vi "open file.vi"(8 "error in (no error)":errorcluster caption="에러 입력(에러 없음)", 10 "file path":path, 11 "Text File 입력":refnum<class "Text File.lvclass">) -> (0 "error out":errorcluster caption="에러 출력", 3 "Text File 출력":refnum<class "Text File.lvclass">)   [LabVIEW 2020, in "Text File.lvclass"]
uses:
  Text File.lvclass
  Haptic IC Class/Haptic IC/Haptic IC.lvclass/Haptic IC.ctl
  Haptic IC Class/Haptic IC/Controls/(Ctrl)IC Type.ctl
  Text File.lvclass/Text File.ctl
  Waveform Obj/Waveform Obj.lvclass/Waveform Obj.ctl
  Accessors/Write Text_File_PWL.vi
  Waveform Obj/Accessors/Write name.vi
  Haptic IC Class/Haptic IC/Accessors/Read ic type.vi
  Waveform Obj/Accessors/Read play mode.vi
  Variables/(Var)System Variables.vi
  Haptic IC Class/Haptic IC/Haptic IC.lvclass
panel:
  in  "TXT_End of LIne":enum16{"EOL (\\r\\n)", "LF (\\n)"}(ring)
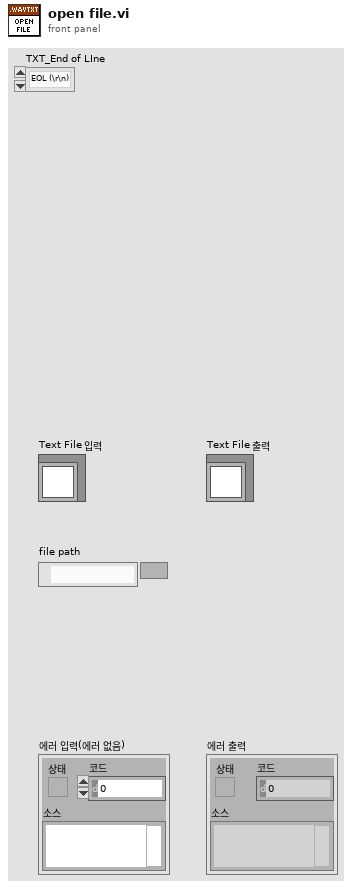
[diagram p1: front panel]
types:
  T1 = cluster{"TXT_Radix":enum16{"BIN", "DEC", "HEX"}, "TXT_Prefix":bool, "TXT_Delimiter":string, "TXT_End of LIne":enum16{"EOL (\\r\\n)", "LF (\\n)"}, "TXT_EOL+Delimiter":bool, "TXT_Number per Line":i32}
  T2 = typedef "Haptic IC.lvclass/(Ctrl)IC Type.ctl" = enum8{"DW7800", "DW7802", "DW7912", "DW7914"}
  T3 = cluster{"Shape":u16, "Ramp":u16, "Amplitude":dbl, "Frequency":dbl, "Cycle":dbl}[]
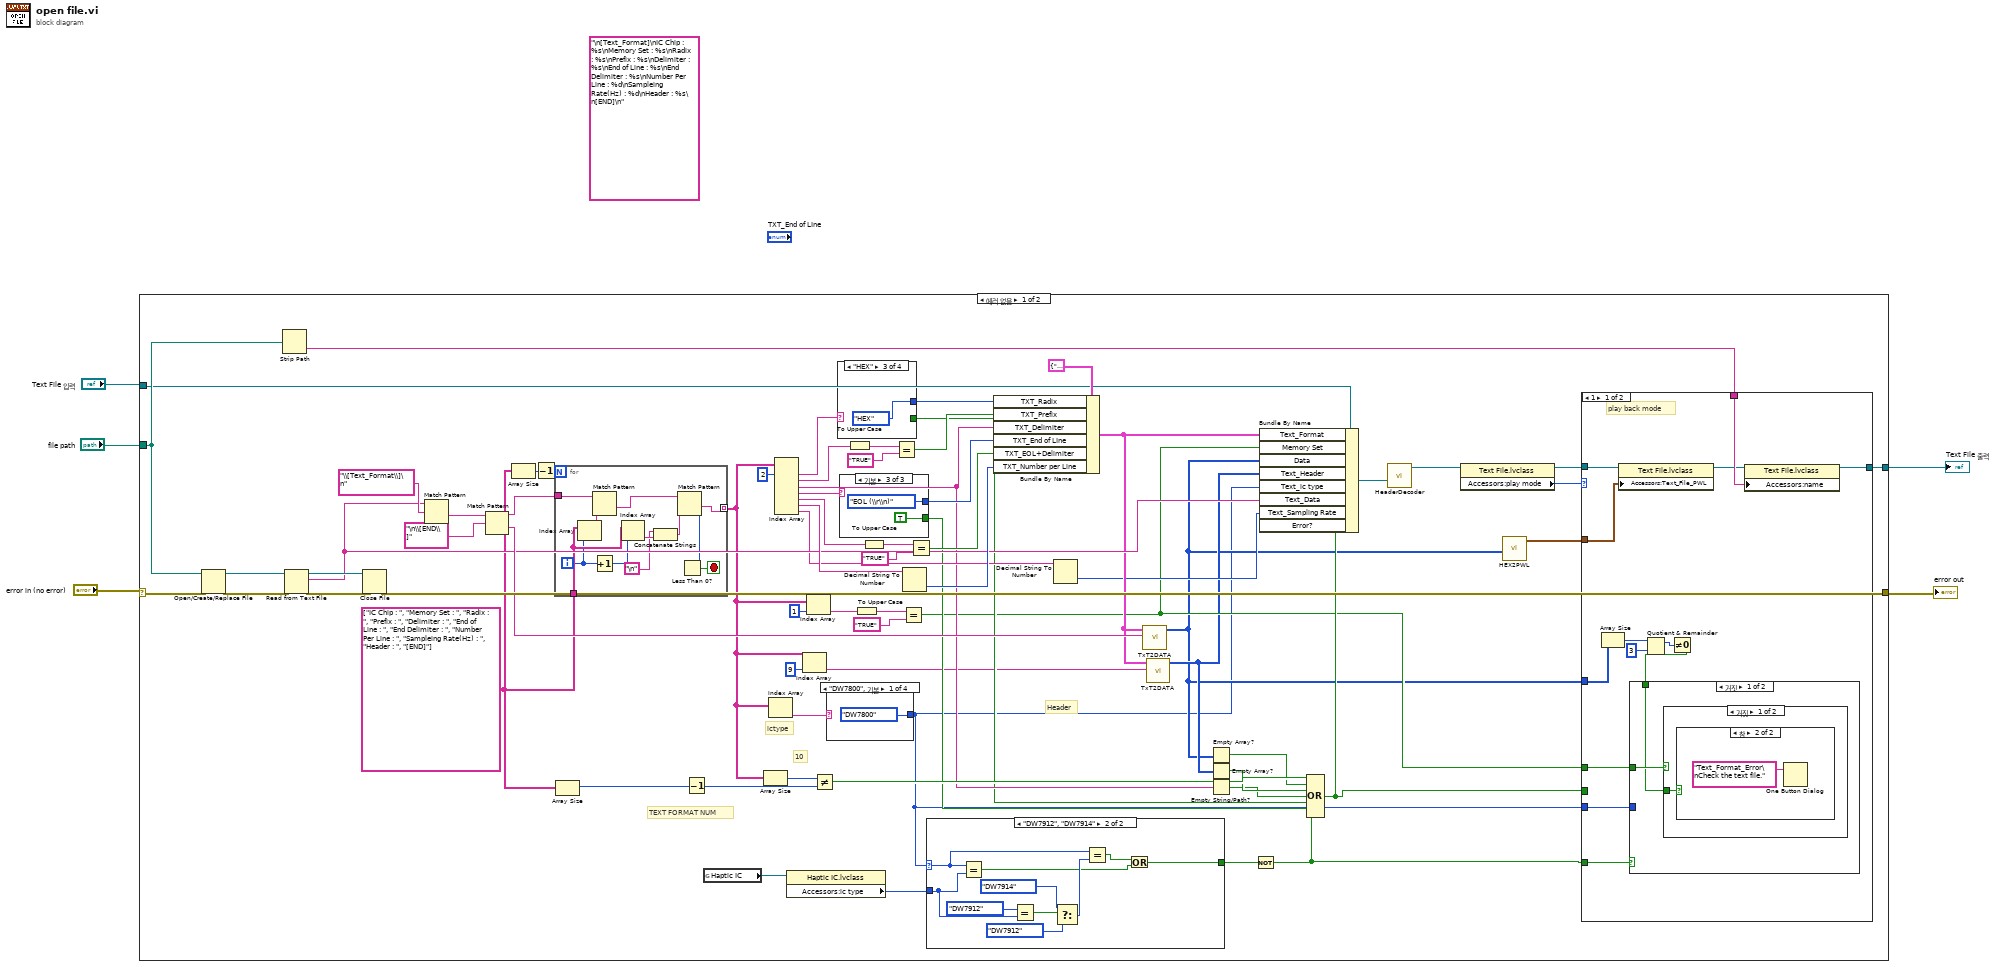
[diagram p0: block diagram]
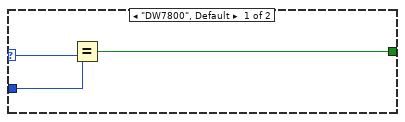
[diagram p2: hidden frame]
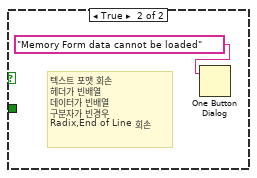
[diagram p4: hidden frame]
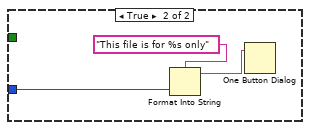
[diagram p5: hidden frame]
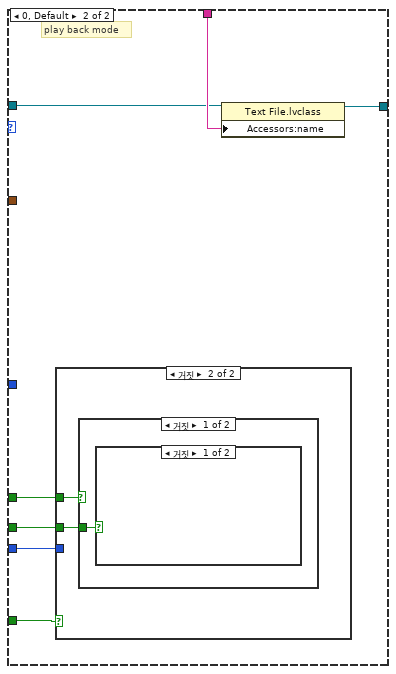
[diagram p6: hidden frame]
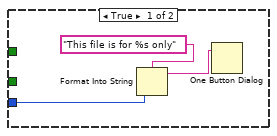
[diagram p7: hidden frame]
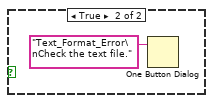
[diagram p8: hidden frame]
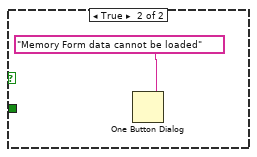
[diagram p9: hidden frame]
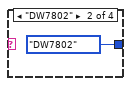
[diagram p10: hidden frame]
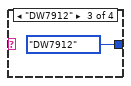
[diagram p11: hidden frame]
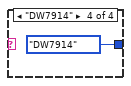
[diagram p12: hidden frame]
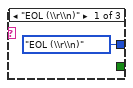
[diagram p13: hidden frame]
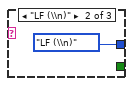
[diagram p14: hidden frame]
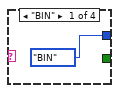
[diagram p15: hidden frame]
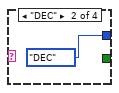
[diagram p16: hidden frame]
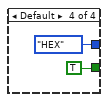
[diagram p17: hidden frame]
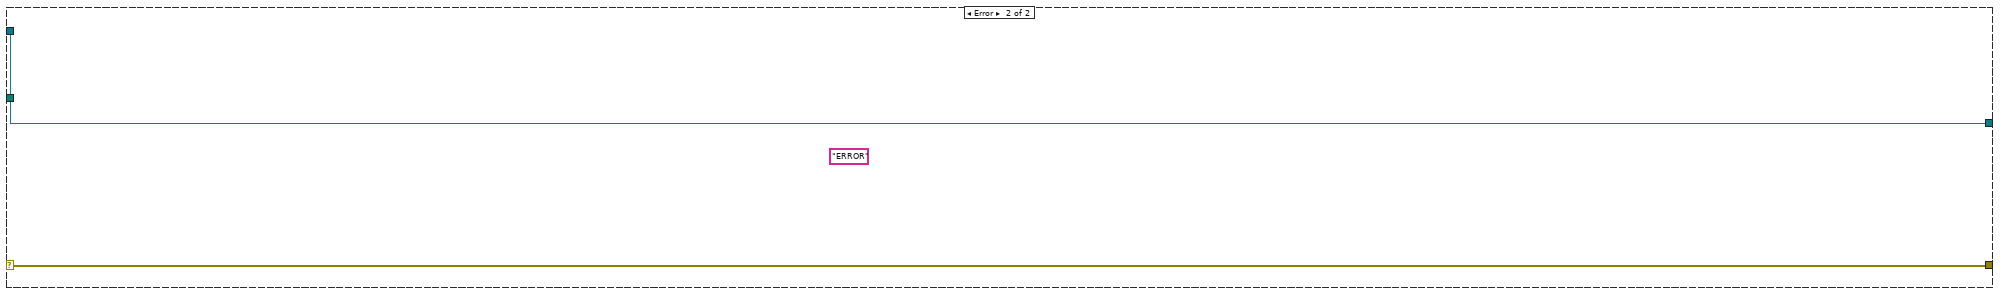
[diagram p18: hidden frame]
diagram:
  (unwired) "\n[Text_Format]\nIC Chip : %s\nMemory Set : %s\nRadix : %s\nPrefix : %s\nDelimiter : %s\nEnd of Line : %s\nEnd Delimiter : %s\nNumber Per Line : %d\nSampleing Rate(Hz) : %d\nHeader : %s\n[END]\n" ("포맷 문자열")
  n1 = case shown="에러 없음" "error in (no error)" {
    selector: "error in (no error)" -> [w75 w151]
    tunnel: [w71 w151] -> w5
    tunnel: [w43 w150] -> w4
    tunnel: "Text File 입력" -> [w42 w150]
    tunnel: "file path" -> [w45 _]
    frame No Error {
      w20 = string[] ["IC Chip : ", "Memory Set : ", "Radix : ", "Prefix : ", "Delimiter : ", "End of Line : ", "End Delimiter : ", "Number Per Line : ", "Sampleing Rate(Hz) : ", "Header : ", "[END]"]
      # "TEXT FORMAT NUM"
      # "10"
      # "ictype"
      # "Header"
      n2 = Open/Create/Replace File(file path (use dialog)=w45, error in=w75) -> (refnum out=w72:refnum<file>, error out=w74:errorcluster)  [unwired: 4 in, 1 out]
      n3 = Strip Path(path=w45) -> (name=w41:string)  [unwired: 1 out]
      n4 = Read from Text File(file (use dialog)=w72, error in=w74) -> (refnum out=w70:refnum<file>, text=w44:string, error out=w73:errorcluster)  [unwired: 2 in, 1 out]
      n5 = Close File(refnum=w70, error in=w73) -> (error out=w71:errorcluster)  [unwired: 1 out]
      n6 = Match Pattern(string=w44, regular expression="\\[Text_Format\\]\n" ("검색 문자열")) -> (after substring=w38:string)  [unwired: 1 in, 3 out]
      n7 = Match Pattern(string=w38, regular expression="\n\\[END\\]" ("정규식")) -> (before substring=w25:string, after substring=w48:string)  [unwired: 1 in, 2 out]
      n8 = Array Size(array=w20) -> (size(s)=w21:i32)
      n9 = Decrement(x=w21) -> (x-1=w17:i32)
      n10 = for {
        N: w17 -> [_]
        tunnel: [w148] -> w23 mode=indexing
        tunnel: w20 -> [w143]
        tunnel: w25 -> [w147]
        i -> [w142]
        stop <- w145 stop-if-true
        n11 = Index Array(array=w143, index=w142) -> (element=w144:string)
        n12 = Match Pattern(string=w147, regular expression=w144) -> (after substring=w149:string)  [unwired: 1 in, 3 out]
        n13 = Increment(x=w142) -> (x+1=w141:i32)
        n14 = Index Array(array=w143, index=w141) -> (element=w140:string)
        n15 = Concatenate Strings("\n", w140) -> (w139:string)
        n16 = Match Pattern(string=w149, regular expression=w139) -> (before substring=w148:string, offset past match=w146:i32)  [unwired: 1 in, 2 out]
        n17 = Less Than 0?(x=w146) -> (x < 0?=w145:bool)
      }
      n18 = Array Size(array=w20) -> (size(s)=w19:i32)
      n19 = Decrement(x=w19) -> (x-1=w18:i32)
      n20 = global read "(Var)System Variables.vi" "Haptic IC"() -> (w10:refnum<class "Haptic IC.lvclass">)
      n21 = Array Size(array=w23) -> (size(s)=w34:i32)
      n22 = Index Array(array=w23) -> (element=w46:string)  [unwired: 1 in]
      n23 = Index Array(array=w23, index #1=2 ("인덱스")) -> (element #1=w63:string, element #2=w60:string, element #3=w29:string, element #4=w59:string, element #5=w56:string, element #6=w55:string, element #7=w36:string)  [unwired: 6 in]
      n24 = property class="Haptic IC.lvclass"(reference=w10) -> ("Accessors:ic type"=w9:T2)  [unwired: 1 in, 2 out]
      n25 = Index Array(array=w23, index=9 ("인덱스")) -> (element=w24:string)
      n26 = Index Array(array=w23, index=1 ("인덱스")) -> (element=w66:string)
      n27 = Not Equal?(x=w34, y=w18) -> (x != y?=w33:bool)
      n28 = case shown="\"DW7800\", 기본" w46 {
        tunnel: [(Ctrl)IC_Type."DW7800" ("Text_ic type") (Ctrl)IC_Type."DW7802" ("Text_ic type") (Ctrl)IC_Type."DW7912" ("Text_ic type") (Ctrl)IC_Type."DW7914" ("Text_ic type")] -> w6
        frame "DW7800", Default {
        }
        frame "DW7802" {
        }
        frame "DW7912" {
        }
        frame "DW7914" {
        }
      }
      n29 = case shown="\"HEX\"" w63 {
        tunnel: [enum16{"BIN", "DEC", "HEX"}."BIN" ("TXT_Radix") enum16{"BIN", "DEC", "HEX"}."DEC" ("TXT_Radix") enum16{"BIN", "DEC", "HEX"}."HEX" ("TXT_Radix") enum16{"BIN", "DEC", "HEX"}."HEX" ("TXT_Radix")] -> w52
        tunnel: [_ _ _ TRUE] -> w28
        frame "BIN" {
        }
        frame "DEC" {
        }
        frame "HEX" {
        }
        frame Default {
        }
      }
      n30 = case shown="기본" w59 {
        tunnel: [enum16{"EOL (\\r\\n)", "LF (\\n)"}."EOL (\\r\\n)" ("TXT_End of LIne") enum16{"EOL (\\r\\n)", "LF (\\n)"}."LF (\\n)" ("TXT_End of LIne") enum16{"EOL (\\r\\n)", "LF (\\n)"}."EOL (\\r\\n)" ("TXT_End of LIne")] -> w49
        tunnel: [_ _ TRUE] -> w26
        frame "EOL (\\r\\n)" {
        }
        frame "LF (\\n)" {
        }
        frame Default {
        }
      }
      n31 = To Upper Case(1:w60) -> (0:w61:string)
      n32 = To Upper Case(1:w66) -> (0:w64:string)
      n33 = To Upper Case(1:w56) -> (0:w57:string)
      n34 = Equal?(x=w61, y="TRUE") -> (x = y?=w51:bool)
      n35 = Equal?(x=w64, y="TRUE") -> (x = y?=w16:bool)
      n36 = Decimal String To Number(string=w55) -> (number=w54:i32)  [unwired: 2 in, 1 out]
      n37 = Equal?(x=w57, y="TRUE") -> (x = y?=w50:bool)
      n38 = case shown="\"DW7912\", \"DW7914\"" w6 {
        selector: w6 -> [w78 w85]
        tunnel: w9 -> [w77 w80]
        tunnel: [w76 w81] -> w8
        frame "DW7800", Default {
          n39 = Equal?(x=w78, y=w77) -> (x = y?=w76:bool)
        }
        frame "DW7912", "DW7914" {
          n40 = Equal?(x=w85, y=w80) -> (x = y?=w82:bool)
          n41 = Equal?(x=(Ctrl)IC_Type."DW7912" ("Accessors:ic type"), y=w80) -> (x = y?=w87:bool)
          n42 = Select(t=(Ctrl)IC_Type."DW7914" ("Accessors:ic type"), s=w87, f=(Ctrl)IC_Type."DW7912" ("Accessors:ic type")) -> (s? t:f=w84:T2)
          n43 = Equal?(x=w85, y=w84) -> (x = y?=w83:bool)
          n44 = Or(x=w83, y=w82) -> (x .or. y?=w81:bool)
        }
      }
      n45 = Bundle By Name(cluster=T1 {"TXT_Radix"=enum."BIN", "TXT_Prefix"=FALSE, "TXT_Delimiter"="", "TXT_End of LIne"=enum."EOL (\\r\\n)", "TXT_EOL+Delimiter"=FALSE, "TXT_Number per Line"=0} ("Text_Format"), "TXT_Radix"=w52, "TXT_Prefix"=w51, "TXT_Delimiter"=w29, "TXT_End of LIne"=w49, "TXT_EOL+Delimiter"=w50, "TXT_Number per Line"=w54) -> (w37:T1)
      n46 = Decimal String To Number(string=w36) -> (number=w35:i32)  [unwired: 2 in, 1 out]
      n47 = call "TxT2DATA.vi"("Text Data"=w48, "Text_Format"=w37) -> ("Data"=w11:i32[])  [unwired: 9 in]
      n48 = call "TxT2DATA.vi"("Text Data"=w24, "Text_Format"=w37) -> ("Data"=w15:i32[])  [unwired: 9 in]
      n49 = Empty Array?(array=w11) -> (empty?=w32:bool)
      n50 = Empty Array?(array=w15) -> (empty?=w31:bool)
      n51 = Empty String/Path?(string/path=w29) -> (empty?=w30:bool)
      n52 = Not(x=w8) -> (.not. x?=w7:bool)
      n53 = Compound Arithmetic op=OR(w33, w32, w31, w30, w28, w26, w7) -> (w27:bool)
      n54 = Bundle By Name(cluster=w42, "Text_Format"=w37, "Memory Set"=w16, "Data"=w11, "Text_Header"=w15, "Text_ic type"=w6, "Text_Data"=w44, "Text_Sampling Rate"=w35, "Error?"=w27) -> (w40:refnum<class "Text File.lvclass">)
      n55 = call "HeaderDecoder.vi"("input class"=w40) -> ("output class"=w39:refnum<class "Text File.lvclass">)  [unwired: 10 in]
      n56 = property class="Text File.lvclass"(reference=w39) -> (reference out=w14:refnum<class "Text File.lvclass">, "Accessors:play mode"=w13:u8)  [unwired: 1 in, 1 out]
      n57 = call "HEX2PWL.vi"("data"=w11) -> ("PWL DATA"=w12:T3)  [unwired: 10 in]
      n58 = case shown="1" w13 {
        tunnel: [w101 w116] -> w43
        tunnel: w41 -> [w100 w115]
        tunnel: w27 -> [_ w114]
        tunnel: w16 -> [w99 w113]
        tunnel: w14 -> [w98 w112]
        tunnel: w12 -> [w96 _]
        tunnel: w11 -> [w95 _]
        tunnel: w7 -> [w89 w111]
        tunnel: w6 -> [w90 w110]
        frame 1 {
          # "play back mode"
          n59 = Array Size(array=w95) -> (size(s)=w94:i32)
          n60 = property class="Text File.lvclass"(reference=w98, "Accessors:Text_File_PWL"=w96) -> (reference out=w97:refnum<class "Text File.lvclass">)  [unwired: 1 in, 1 out]
          n61 = Quotient & Remainder(x=w94, y=3) -> (x-y*floor(x/y)=w92:i32)  [unwired: 1 out]
          n62 = Not Equal To 0?(x=w92) -> (x != 0?=w91:bool)
          n63 = case shown="거짓" w89 {
            tunnel: w99 -> [w103 _]
            tunnel: w91 -> [w102 _]
            tunnel: w90 -> [_ w107]
            frame False {
              n64 = case shown="거짓" w103 {
                tunnel: w102 -> [w104 _]
                frame False {
                  n65 = case shown="참" w104 {
                    frame False {
                    }
                    frame True {
                      n66 = One Button Dialog(message="Text_Format_Error\nCheck the text file." ("메시지")) -> ()  [unwired: 1 in, 1 out]
                    }
                  }
                }
                frame True {
                  # "텍스트 포맷 회손\n헤더가 빈배열\n데이터가 빈배열\n구분자가 빈경우\nRadix,End of Line 회손"
                  n67 = One Button Dialog(message="Memory Form data cannot be loaded" ("메시지")) -> ()  [unwired: 1 in, 1 out]
                }
              }
            }
            frame True {
              n68 = Format Into String(format string="This file is for %s only" ("포맷 문자열"), w107) -> (resulting string=w109:string)  [unwired: 2 in, 1 out]
              n69 = One Button Dialog(message=w109) -> ()  [unwired: 1 in, 1 out]
            }
          }
          n70 = property class="Text File.lvclass"(reference=w97, "Accessors:name"=w100) -> (reference out=w101:refnum<class "Text File.lvclass">)  [unwired: 1 in, 1 out]
        }
        frame 0, Default {
          # "play back mode"
          n71 = case shown="거짓" w111 {
            tunnel: w114 -> [_ w121]
            tunnel: w113 -> [_ w120]
            tunnel: w110 -> [w117 _]
            frame True {
              n72 = Format Into String(format string="This file is for %s only" ("포맷 문자열"), w117) -> (resulting string=w119:string)  [unwired: 2 in, 1 out]
              n73 = One Button Dialog(message=w119) -> ()  [unwired: 1 in, 1 out]
            }
            frame False {
              n74 = case shown="거짓" w120 {
                tunnel: w121 -> [w122 _]
                frame False {
                  n75 = case shown="거짓" w122 {
                    frame False {
                    }
                    frame True {
                      n76 = One Button Dialog(message="Text_Format_Error\nCheck the text file." ("메시지")) -> ()  [unwired: 1 in, 1 out]
                    }
                  }
                }
                frame True {
                  n77 = One Button Dialog(message="Memory Form data cannot be loaded" ("메시지")) -> ()  [unwired: 1 in, 1 out]
                }
              }
            }
          }
          n78 = property class="Text File.lvclass"(reference=w112, "Accessors:name"=w115) -> (reference out=w116:refnum<class "Text File.lvclass">)  [unwired: 1 in, 1 out]
        }
      }
    }
    frame Error {
      (unwired) "ERROR"
    }
  }
  "error out" <- w5
  "Text File 출력" <- w4
